vi "StartCAN.1.vi"(11 "CAN Interface":refnum<k21>="CAN1") -> (0 "error out":errorcluster, 1 "Tester Write Session out":refnum<k21>, 2 "Read Session out":refnum<k21>, 3 "DSC Write Session out":refnum<k21>)   [LabVIEW 2018]
uses:
  <vilib>/xnet/xnet.llb/XNET CAN Comm State.ctl
  <vilib>/xnet/xnet.llb/XNET Control Scope.ctl
  <vilib>/xnet/xnet.llb/XNET Frame CAN.ctl
  <vilib>/xnet/xnet.llb/XNET Frame Type CAN.ctl
  <vilib>/xnet/xnet.llb/XNET Create Session (Frame Input Queued).vi
  <vilib>/xnet/xnet.llb/XNET Create Session (Frame Output Single-point).vi
  <vilib>/xnet/xnet.llb/XNET Read (State CAN Comm).vi
  <vilib>/xnet/xnet.llb/XNET Wait (Interface Communicating).vi
  <resource>/objmgr/xnet.rc
  <vilib>/xnet/xnet.llb/XNET Write (Frame CAN).vi
panel:
  in  "error in (no error)":errorcluster
  out "TesterPresentSession":refnum<k21>
  out "CAN:I/O Mode":u32(ring) items=["CAN 2.0", "CAN FD", "CAN FD+BRS"]
  out "Protocol":u32(ring) items=["CAN", "FlexRay", "LIN"]
  out "CAN:Transceiver Capability":u32(ring) items=["HS"=0, "LS"=1, "XS"=3, "XS (HS/LS)"=4]
  out "Interface:CAN:Transceiver State":u32(ring) items=["Normal", "Sleep", "Single Wire Wakeup", "Single Wire High-Speed"]
  out "Interface:CAN:Transceiver State 2":u32(ring) items=["Normal", "Sleep", "Single Wire Wakeup", "Single Wire High-Speed"]
  out "Interface:CAN:Transceiver State 3":u32(ring) items=["Normal", "Sleep", "Single Wire Wakeup", "Single Wire High-Speed"]
  out "CAN:Termination Capability":u32(ring) items=["No", "Yes"]
  out "Array":T1[](array[typedef]) items=["Error Active", "Error Passive", "Bus Off", "Init"]
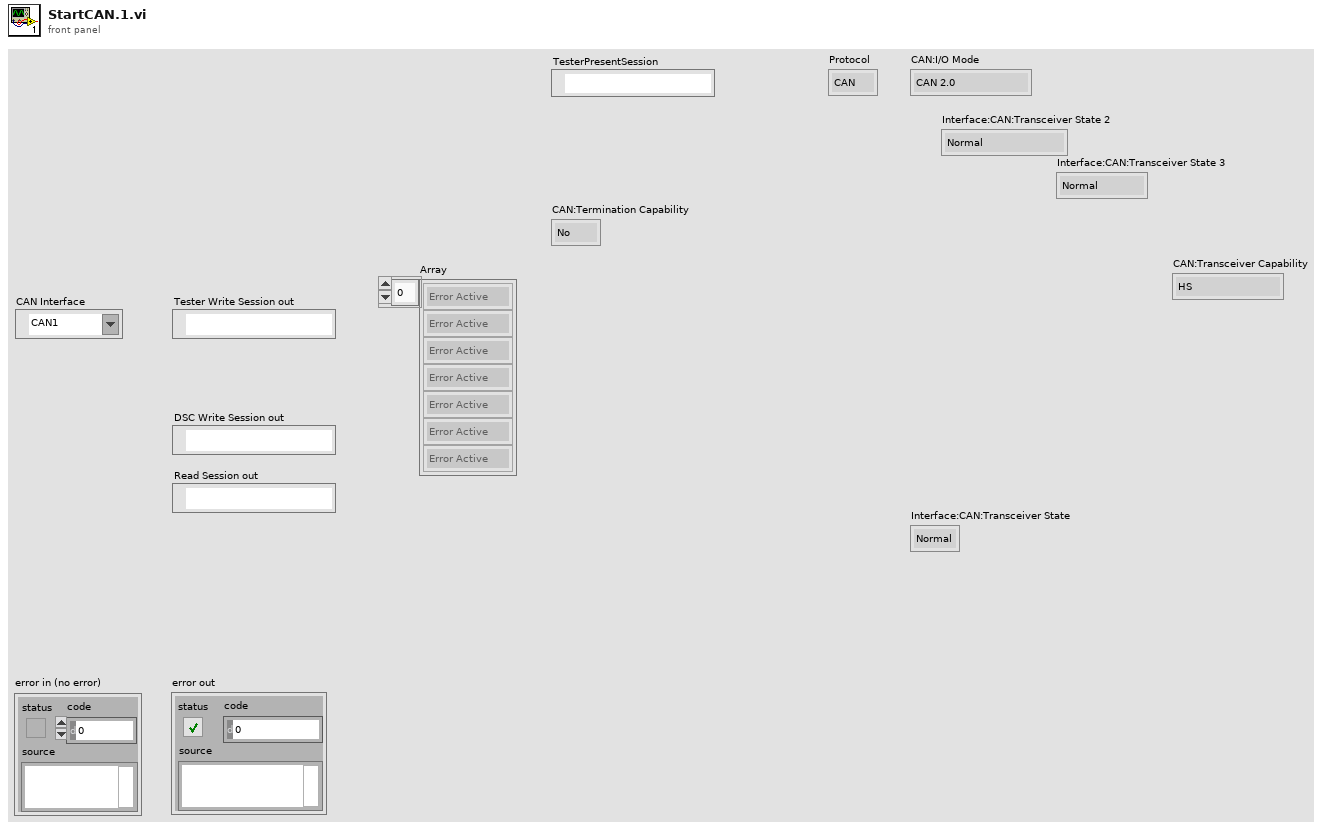
[diagram p1: front panel]
types:
  T1 = typedef "XNET CAN Comm State.ctl" = u8
  T2 = cluster{"Comment":string, "Default Payload":u8[], "Identifier":u32, "Name (Short)":string, "Payload Length":u32, "PDU_Mapping":cluster{"PDU":string, "Start Bit":u32, "Update Bit":i32}[], "CAN:Extended Identifier?":bool, "CAN:Timing Type":u32, "CAN:Transmit Time":dbl, "CAN:I/O Mode":u32}
  T3 = typedef "XNET Frame CAN.ctl" = cluster{"timestamp":timestamp, "payload":u8[], "identifier":u32, "type":T4, "extended?":bool, "echo?":bool}
  T4 = typedef "XNET Frame Type CAN.ctl" = u8
  T5 = typedef "XNET Control Scope.ctl" = u32
  T6 = typedef "XNET CAN Comm.ctl" = cluster{"fault code":i32, "fault?":bool, "communication state":T1, "last error":T7, "receive error counter":u8, "transmit error counter":u8, "transceiver error?":bool, "sleep?":bool}
  T7 = typedef "XNET CAN Last Err.ctl" = u8
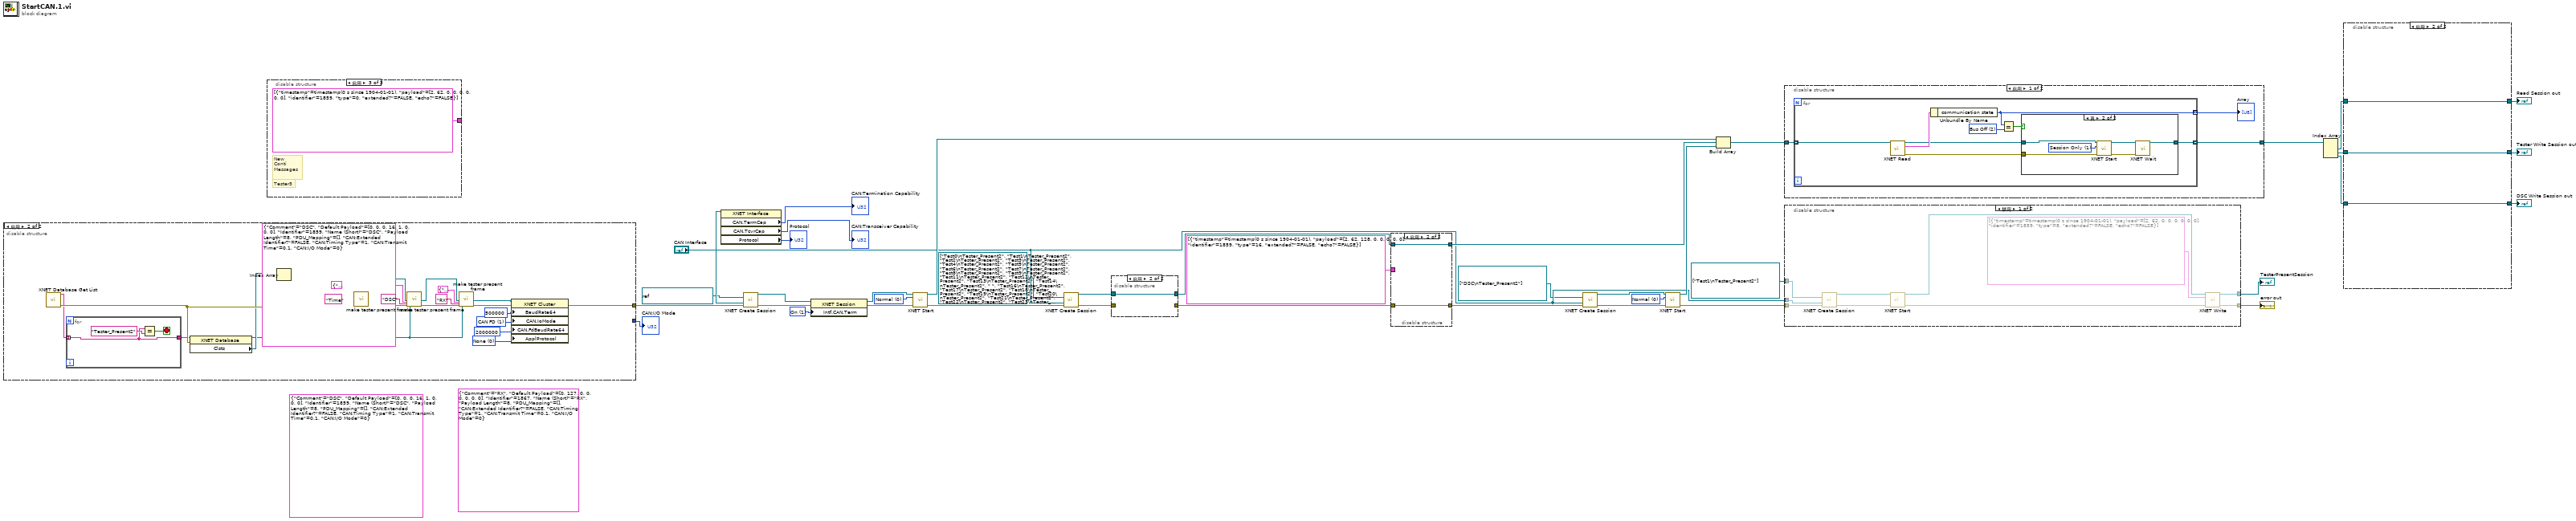
[diagram p0: block diagram]
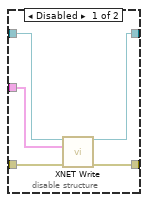
[diagram p2: hidden frame]
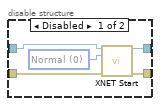
[diagram p3: hidden frame]
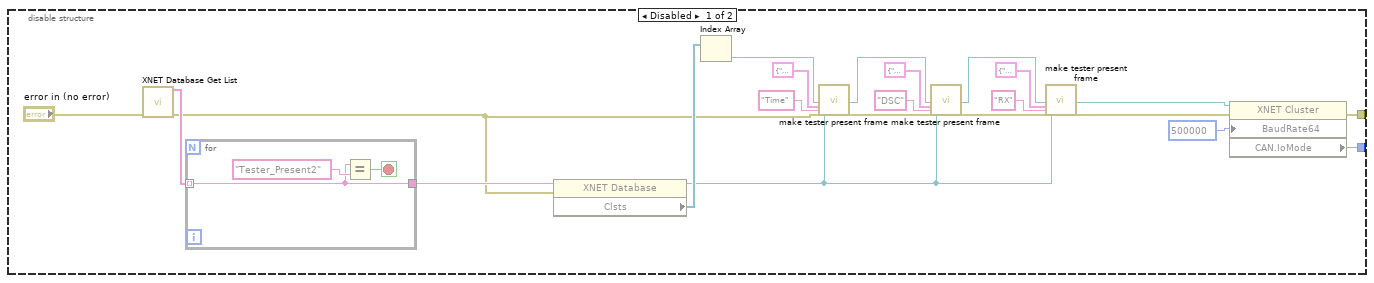
[diagram p4: hidden frame]
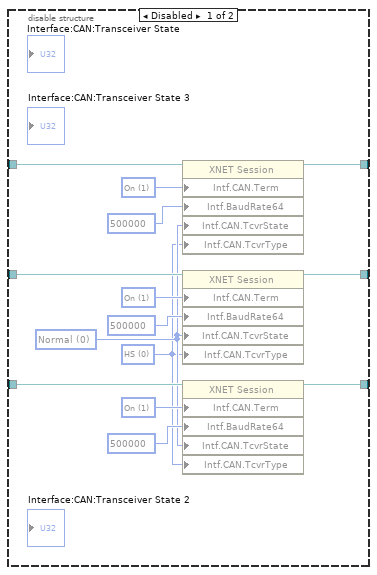
[diagram p6: hidden frame]
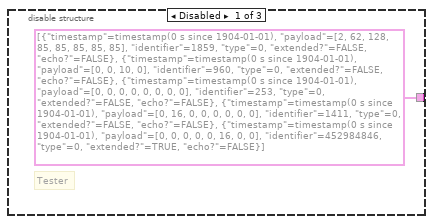
[diagram p9: hidden frame]
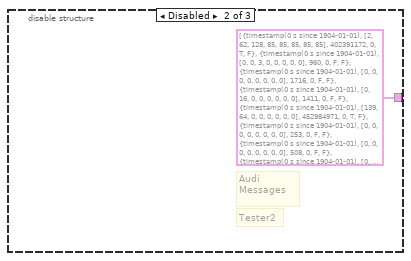
[diagram p10: hidden frame]
diagram:
  (unwired) T2 {"Comment"="DSC", "Default Payload"=[0, 0, 0, 16, 1, 0, 0, 0], "Identifier"=1859, "Name (Short)"="DSC", "Payload Length"=8, "PDU_Mapping"=[], "CAN:Extended Identifier?"=FALSE, "CAN:Timing Type"=1, "CAN:Transmit Time"=0.1, "CAN:I/O Mode"=0} ("New Frame Properties")
  (unwired) T2 {"Comment"="RX", "Default Payload"=[0, 127, 0, 0, 0, 0, 0, 0], "Identifier"=1867, "Name (Short)"="RX", "Payload Length"=8, "PDU_Mapping"=[], "CAN:Extended Identifier?"=FALSE, "CAN:Timing Type"=1, "CAN:Transmit Time"=0.1, "CAN:I/O Mode"=0} ("New Frame Properties")
  w11 = u32 1 items=["Off", "On"] ("Interface:CAN:Termination")
  w29 = T5 0 items=["Normal", "Session Only", "Interface Only", "Session Only Blocking"] ("scope (normal)")
  w30 = T5 0 items=["Normal", "Session Only", "Interface Only", "Session Only Blocking"] ("scope (normal)")
  n1 = disable-structure shown="启用" {
    disable-tunnel: [w60 w69] -> w40
    disable-tunnel: [w41 _] -> w15
    frame Disabled {
      n2 = call <vilib>:"XNET Database Get List.vi"("error in (no error)"="error in (no error)") -> ("array of alias"=w50:string[], "error out"=w46:errorcluster)  [unwired: 12 in, 1 out]
      n3 = for {
        tunnel: w50 -> [w63] mode=indexing
        tunnel: [w63] -> w49
        stop <- w64 stop-if-true
        n4 = Equal?(x=w63, y="Tester_Present2") -> (x = y?=w64:bool)
      }
      n5 = property class="XNET Database"(reference=w49, error in=w46) -> (reference out=w42:refnum<k21>, "Clsts"=w61:refnum<k21>[])  [unwired: 1 out]
      n6 = Index Array(array=w61) -> (element=w44:refnum<k21>)  [unwired: 1 in]
      n7 = call "make tester present frame.vi"("Cluster::"=w44, "New Frame Properties"=T2 {"Comment"="DSC", "Default Payload"=[0, 0, 0, 0, 0, 0, 0, 0], "Identifier"=1714, "Name (Short)"="Time", "Payload Length"=8, "PDU_Mapping"=[], "CAN:Extended Identifier?"=FALSE, "CAN:Timing Type"=0, "CAN:Transmit Time"=0.001, "CAN:I/O Mode"=0}, "frame name"="Time", "error in (no error)"=w46, "database in"=w42) -> ("target cluster out"=w43:refnum<k21>, "error out"=w45:errorcluster)  [unwired: 21 in]
      n8 = call "make tester present frame.vi"("Cluster::"=w43, "New Frame Properties"=T2 {"Comment"="DSC", "Default Payload"=[0, 0, 0, 0, 0, 0, 0, 0], "Identifier"=402391172, "Name (Short)"="DSC", "Payload Length"=8, "PDU_Mapping"=[], "CAN:Extended Identifier?"=TRUE, "CAN:Timing Type"=1, "CAN:Transmit Time"=0.001, "CAN:I/O Mode"=0}, "frame name"="DSC", "error in (no error)"=w45, "database in"=w42) -> ("target cluster out"=w59:refnum<k21>, "error out"=w58:errorcluster)  [unwired: 21 in]
      n9 = call "make tester present frame.vi"("Cluster::"=w59, "New Frame Properties"=T2 {"Comment"="RX", "Default Payload"=[0, 127, 0, 0, 0, 0, 0, 0], "Identifier"=402522244, "Name (Short)"="RX", "Payload Length"=8, "PDU_Mapping"=[], "CAN:Extended Identifier?"=TRUE, "CAN:Timing Type"=1, "CAN:Transmit Time"=0.001, "CAN:I/O Mode"=0}, "frame name"="RX", "error in (no error)"=w58, "database in"=w42) -> ("target cluster out"=w52:refnum<k21>, "error out"=w51:errorcluster)  [unwired: 21 in]
      n10 = property class="XNET Cluster"(reference=w52, error in=w51, "BaudRate64"=u64 500000 ("64bit Baud Rate")) -> (error out=w60:errorcluster, "CAN.IoMode"=w41:u32)  [unwired: 1 out]
    }
    frame Enabled {
      w66 = u32 0 items=["None", "J1939"] ("Application Protocol")
      w68 = u32 1 items=["CAN 2.0", "CAN FD", "CAN FD+BRS"] ("CAN:I/O Mode")
      n11 = call <vilib>:"XNET Database Get List.vi"() -> ("array of alias"=w85:string[], "error out"=w86:errorcluster)  [unwired: 13 in, 1 out]
      n12 = for {
        tunnel: w85 -> [w89] mode=indexing
        tunnel: [w89] -> w72
        stop <- w90 stop-if-true
        n13 = Equal?(x=w89, y="Tester_Present2") -> (x = y?=w90:bool)
      }
      n14 = property class="XNET Database"(reference=w72, error in=w86) -> (reference out=w71:refnum<k21>, "Clsts"=w73:refnum<k21>[])  [unwired: 1 out]
      n15 = Index Array(array=w73) -> (element=w88:refnum<k21>)  [unwired: 1 in]
      n16 = call "make tester present frame.vi"("Cluster::"=w88, "New Frame Properties"=T2 {"Comment"="Time", "Default Payload"=[0, 0, 0, 0, 0, 0, 0, 0], "Identifier"=1859, "Name (Short)"="Time", "Payload Length"=8, "PDU_Mapping"=[], "CAN:Extended Identifier?"=FALSE, "CAN:Timing Type"=0, "CAN:Transmit Time"=0.1, "CAN:I/O Mode"=0}, "frame name"="Time", "error in (no error)"=w86, "database in"=w71) -> ("target cluster out"=w70:refnum<k21>, "error out"=w87:errorcluster)  [unwired: 21 in]
      n17 = call "make tester present frame.vi"("Cluster::"=w70, "New Frame Properties"=T2 {"Comment"="DSC", "Default Payload"=[0, 0, 0, 16, 1, 0, 0, 0], "Identifier"=1859, "Name (Short)"="DSC", "Payload Length"=8, "PDU_Mapping"=[], "CAN:Extended Identifier?"=FALSE, "CAN:Timing Type"=1, "CAN:Transmit Time"=0.1, "CAN:I/O Mode"=0}, "frame name"="DSC", "error in (no error)"=w87, "database in"=w71) -> ("target cluster out"=w81:refnum<k21>, "error out"=w82:errorcluster)  [unwired: 21 in]
      n18 = call "make tester present frame.vi"("Cluster::"=w81, "New Frame Properties"=T2 {"Comment"="RX", "Default Payload"=[0, 0, 0, 0, 0, 0, 0, 0], "Identifier"=1867, "Name (Short)"="RX", "Payload Length"=8, "PDU_Mapping"=[], "CAN:Extended Identifier?"=FALSE, "CAN:Timing Type"=1, "CAN:Transmit Time"=0.001, "CAN:I/O Mode"=1}, "frame name"="RX", "error in (no error)"=w82, "database in"=w71) -> ("target cluster out"=w83:refnum<k21>, "error out"=w84:errorcluster)  [unwired: 21 in]
      n19 = property class="XNET Cluster"(reference=w83, error in=w84, "BaudRate64"=u64 500000 ("64bit Baud Rate"), "CAN.IoMode"=w68, "CAN.FdBaudRate64"=u64 2000000 ("CAN:64bit FD Baud Rate"), "ApplProtocol"=w66) -> (error out=w69:errorcluster)  [unwired: 1 out]
    }
  }
  "CAN:I/O Mode" <- w15
  n20 = disable-structure shown="启用" {
    disable-tunnel: [T3[] [{"timestamp"=timestamp(0 s since 1904-01-01), "payload"=[2, 62, 128, 85, 85, 85, 85, 85], "identifier"=1859, "type"=0, "extended?"=FALSE, "echo?"=FALSE}, {"timestamp"=timestamp(0 s since 1904-01-01), "payload"=[0, 0, 10, 0], "identifier"=960, "type"=0, "extended?"=FALSE, "echo?"=FALSE}, {"timestamp"=timestamp(0 s since 1904-01-01), "payload"=[0, 0, 0, 0, 0, 0, 0, 0], "identifier"=253, "type"=0, "extended?"=FALSE, "echo?"=FALSE}, {"timestamp"=timestamp(0 s since 1904-01-01), "payload"=[0, 16, 0, 0, 0, 0, 0, 0], "identifier"=1411, "type"=0, "extended?"=FALSE, "echo?"=FALSE}, {"timestamp"=timestamp(0 s since 1904-01-01), "payload"=[0, 0, 0, 0, 0, 16, 0, 0], "identifier"=452984846, "type"=0, "extended?"=TRUE, "echo?"=FALSE}] ("data") T3[] [{"timestamp"=timestamp(0 s since 1904-01-01), "payload"=[2, 62, 128, 85, 85, 85, 85, 85], "identifier"=402391172, "type"=0, "extended?"=TRUE, "echo?"=FALSE}, {"timestamp"=timestamp(0 s since 1904-01-01), "payload"=[0, 0, 3, 0, 0, 0, 0, 0], "identifier"=960, "type"=0, "extended?"=FALSE, "echo?"=FALSE}, {"timestamp"=timestamp(0 s since 1904-01-01), "payload"=[0, 0, 0, 0, 0, 0, 0, 0], "identifier"=1716, "type"=0, "extended?"=FALSE, "echo?"=FALSE}, {"timestamp"=timestamp(0 s since 1904-01-01), "payload"=[0, 16, 0, 0, 0, 0, 0, 0], "identifier"=1411, "type"=0, "extended?"=FALSE, "echo?"=FALSE}, {"timestamp"=timestamp(0 s since 1904-01-01), "payload"=[139, 64, 0, 0, 0, 0, 0, 0], "identifier"=452984971, "type"=0, "extended?"=TRUE, "echo?"=FALSE}, {"timestamp"=timestamp(0 s since 1904-01-01), "payload"=[0, 0, 0, 0, 0, 0, 0, 0], "identifier"=253, "type"=0, "extended?"=FALSE, "echo?"=FALSE}, {"timestamp"=timestamp(0 s since 1904-01-01), "payload"=[0, 0, 0, 0, 0, 0, 0, 0], "identifier"=508, "type"=0, "extended?"=FALSE, "echo?"=FALSE}, {"timestamp"=timestamp(0 s since 1904-01-01), "payload"=[0, 0, 0, 0, 150, 0, 0, 0], "identifier"=1646, "type"=0, "extended?"=FALSE, "echo?"=FALSE}, {"timestamp"=timestamp(0 s since 1904-01-01), "payload"=[0, 0, 0, 0, 0, 0, 0, 150], "identifier"=1719, "type"=0, "extended?"=FALSE, "echo?"=FALSE}, {"timestamp"=timestamp(0 s since 1904-01-01), "payload"=[0, 0, 4, 0, 0, 0, 0, 0], "identifier"=958, "type"=0, "extended?"=FALSE, "echo?"=FALSE}, {"timestamp"=timestamp(0 s since 1904-01-01), "payload"=[0, 0, 0, 0, 0, 0, 0, 0], "identifier"=1635, "type"=0, "extended?"=FALSE, "echo?"=FALSE}, {"timestamp"=timestamp(0 s since 1904-01-01), "payload"=[0, 0, 0, 0, 0, 0, 0, 0], "identifier"=319, "type"=0, "extended?"=FALSE, "echo?"=FALSE}, {"timestamp"=timestamp(0 s since 1904-01-01), "payload"=[0, 0, 0, 0, 0, 0, 0, 0], "identifier"=1616, "type"=0, "extended?"=FALSE, "echo?"=FALSE}, {"timestamp"=timestamp(0 s since 1904-01-01), "payload"=[0, 12, 0, 0, 0, 0, 0, 0], "identifier"=1413, "type"=0, "extended?"=FALSE, "echo?"=FALSE}, {"timestamp"=timestamp(0 s since 1904-01-01), "payload"=[0, 0, 0, 0, 0, 0, 0, 0], "identifier"=1462, "type"=0, "extended?"=FALSE, "echo?"=FALSE}, {"timestamp"=timestamp(0 s since 1904-01-01), "payload"=[16, 64, 0, 0, 0, 16, 0, 0], "identifier"=452984848, "type"=0, "extended?"=TRUE, "echo?"=FALSE}, {"timestamp"=timestamp(0 s since 1904-01-01), "payload"=[0, 0, 0, 0, 0, 0, 0, 0], "identifier"=976, "type"=0, "extended?"=FALSE, "echo?"=FALSE}, {"timestamp"=timestamp(0 s since 1904-01-01), "payload"=[0, 0, 0, 0, 0, 0, 0, 0], "identifier"=974, "type"=0, "extended?"=FALSE, "echo?"=FALSE}, {"timestamp"=timestamp(0 s since 1904-01-01), "payload"=[74, 64, 0, 0, 0, 0, 0, 0], "identifier"=452984906, "type"=0, "extended?"=TRUE, "echo?"=FALSE}, {"timestamp"=timestamp(0 s since 1904-01-01), "payload"=[0, 0, 0, 0, 0, 0, 0, 0], "identifier"=977, "type"=0, "extended?"=FALSE, "echo?"=FALSE}, {"timestamp"=timestamp(0 s since 1904-01-01), "payload"=[0, 0, 0, 0, 0, 0, 0, 0], "identifier"=975, "type"=0, "extended?"=FALSE, "echo?"=FALSE}, {"timestamp"=timestamp(0 s since 1904-01-01), "payload"=[75, 64, 0, 0, 0, 0, 0, 0], "identifier"=452984907, "type"=0, "extended?"=TRUE, "echo?"=FALSE}] ("Array 3") T3[] [{"timestamp"=timestamp(0 s since 1904-01-01), "payload"=[2, 62, 0, 0, 0, 0, 0, 0], "identifier"=1859, "type"=0, "extended?"=FALSE, "echo?"=FALSE}] ("data")] -> _
    frame Disabled {
      # "Tester"
    }
    frame Disabled {
      # "Tester2"
      # "Audi\nMessages"
    }
    frame Enabled {
      # "Tester3"
      # "New\nConti\nMessages"
    }
  }
  n21 = property class="XNET Interface"(reference="CAN Interface") -> ("CAN.TermCap"=→"CAN:Termination Capability":u32, "CAN.TcvrCap"=→"CAN:Transceiver Capability":u32, "Protocol"=→"Protocol":u32)  [unwired: 1 in, 2 out]
  n22 = call-poly <vilib>:"XNET Create Session.vi"("frame"=refnum<k21> "RX\nTester_Present2" ("XNET Frame"), "interface"="CAN Interface", "error in (no error)"=w40) -> ("session out"=w14:refnum<k21>, "error out"=w12:errorcluster)  [unwired: 11 in]
  n23 = property class="XNET Session"(reference=w14, error in=w12, "Intf.CAN.Term"=w11) -> (reference out=w13:refnum<k21>, error out=w10:errorcluster)
  n24 = call <vilib>:"XNET Start.vi"("session in"=w13, "scope (normal)"=w30, "error in (no error)"=w10) -> ("session out"=w37:refnum<k21>, "error out"=w32:errorcluster)  [unwired: 11 in]
  n25 = call-poly <vilib>:"XNET Create Session.vi"("frame list"=refnum<k21>[] ["Test0\nTester_Present2", "Test1\nTester_Present2", "Test2\nTester_Present2", "Test3\nTester_Present2", "Test4\nTester_Present2", "Test5\nTester_Present2", "Test6\nTester_Present2", "Test7\nTester_Present2", "Test8\nTester_Present2", "Test9\nTester_Present2", "Test11\nTester_Present2", "Test12\nTester_Present2", "Test13\nTester_Present2", "Test14\nTester_Present2", " ", "Test16\nTester_Present2", "Test17\nTester_Present2", "Test18\nTester_Present2", "Test19\nTester_Present2", "Test20\nTester_Present2", "Test21\nTester_Present2", "Test22\nTester_Present2", "Test23\nTester_Present2", "Test24\nTester_Present2", "Test25\nTester_Present2", "Test26\nTester_Present2", "Test27\nTester_Present2"] ("Frames"), "interface"="CAN Interface", "error in (no error)"=w32) -> ("session out"=w27:refnum<k21>, "error out"=w28:errorcluster)  [unwired: 11 in]
  n26 = disable-structure shown="启用" {
    disable-tunnel: [w99 w100] -> w39
    disable-tunnel: [w98 _] -> w38
    disable-tunnel: w28 -> [w96 _]
    disable-tunnel: w27 -> [w95 w100]
    frame Disabled {
      w97 = T5 0 items=["Normal", "Session Only", "Interface Only", "Session Only Blocking"] ("scope (normal)")
      n27 = call <vilib>:"XNET Start.vi"("session in"=w95, "scope (normal)"=w97, "error in (no error)"=w96) -> ("session out"=w99:refnum<k21>, "error out"=w98:errorcluster)  [unwired: 11 in]
    }
    frame Enabled {
    }
  }
  n28 = disable-structure shown="启用" {
    disable-tunnel: w39 -> [w105 w106]
    disable-tunnel: w38 -> [w104 w107]
    disable-tunnel: [w103 w106] -> w36
    disable-tunnel: [w102 w107] -> w31
    disable-tunnel: T3[] [{"timestamp"=timestamp(0 s since 1904-01-01), "payload"=[2, 62, 128, 0, 0, 0, 0, 0], "identifier"=1859, "type"=16, "extended?"=FALSE, "echo?"=FALSE}] ("data") -> [w101 _]
    frame Disabled {
      n29 = call-poly <vilib>:"XNET Write.vi"("session in"=w105, "data"=w101, "error in (no error)"=w104) -> ("session out"=w103:refnum<k21>, "error out"=w102:errorcluster)  [unwired: 11 in]
    }
    frame Enabled {
    }
  }
  n30 = call-poly <vilib>:"XNET Create Session.vi"("frame list"=refnum<k21>[] ["DSC\nTester_Present2"] ("Frames"), "interface"="CAN Interface", "error in (no error)"=w31) -> ("session out"=w26:refnum<k21>, "error out"=w25:errorcluster)  [unwired: 11 in]
  n31 = call <vilib>:"XNET Start.vi"("session in"=w26, "scope (normal)"=w29, "error in (no error)"=w25) -> ("session out"=w35:refnum<k21>, "error out"=w6:errorcluster)  [unwired: 11 in]
  n32 = Build Array(w37, w36, w35) -> (w34:refnum<k21>[])
  n33 = disable-structure shown="启用" {
    disable-tunnel: w34 -> [w110 w126]
    disable-tunnel: [w108 w126] -> w33
    frame Enabled {
      n34 = for {
        tunnel: w110 -> [w117] mode=indexing
        tunnel: [w112] -> w109 mode=indexing
        tunnel: [w111] -> w108 mode=indexing
        w116 = T1 2 items=["Error Active", "Error Passive", "Bus Off", "Init"] ("y")
        n35 = call-poly <vilib>:"XNET Read.vi"("session in"=w117) -> ("session out"=w114:refnum<k21>, "CAN comm"=w118:T6, "error out"=w113:errorcluster)  [unwired: 12 in]
        n36 = Unbundle By Name(w118) -> ("communication state"=w112:T1)
        n37 = Equal?(x=w112, y=w116) -> (x = y?=w115:bool)
        n38 = case shown="真" w115 {
          tunnel: w114 -> [w119 w125]
          tunnel: w113 -> [_ w123]
          tunnel: [w119 w120] -> w111
          frame False {
          }
          frame True {
            w121 = T5 1 items=["Normal", "Session Only", "Interface Only", "Session Only Blocking"] ("scope (normal)")
            n39 = call <vilib>:"XNET Start.vi"("session in"=w125, "scope (normal)"=w121, "error in (no error)"=w123) -> ("session out"=w124:refnum<k21>, "error out"=w122:errorcluster)  [unwired: 11 in]
            n40 = call-poly <vilib>:"XNET Wait.vi"("session in"=w124, "error in (no error)"=w122) -> ("session out"=w120:refnum<k21>)  [unwired: 12 in, 1 out]
          }
        }
      }
      "Array" <- w109
    }
    frame Disabled {
    }
  }
  n41 = disable-structure shown="禁用" {
    disable-tunnel: "CAN Interface" -> [w136 _]
    disable-tunnel: [w128 _] -> w8
    disable-tunnel: [w129 _] -> w7
    disable-tunnel: refnum<k21>[] ["Test1\nTester_Present2"] ("Frames") -> [w135 _]
    disable-tunnel: w6 -> [w132 _]
    frame Disabled {
      n42 = call-poly <vilib>:"XNET Create Session.vi"("frame list"=w135, "interface"=w136, "error in (no error)"=w132) -> ("session out"=w134:refnum<k21>, "error out"=w133:errorcluster)  [unwired: 11 in]
      n43 = call <vilib>:"XNET Start.vi"("session in"=w134, "error in (no error)"=w133) -> ("session out"=w131:refnum<k21>, "error out"=w130:errorcluster)  [unwired: 12 in]
      n44 = call-poly <vilib>:"XNET Write.vi"("session in"=w131, "data"=T3[] [{"timestamp"=timestamp(0 s since 1904-01-01), "payload"=[2, 62, 0, 0, 0, 0, 0, 0], "identifier"=1859, "type"=8, "extended?"=FALSE, "echo?"=FALSE}], "error in (no error)"=w130) -> ("session out"=w128:refnum<k21>, "error out"=w129:errorcluster)  [unwired: 11 in]
    }
    frame Enabled {
    }
  }
  "error out" <- w7
  "TesterPresentSession" <- w8
  n45 = Index Array(array=w33) -> (element #1=w23:refnum<k21>, element #2=w21:refnum<k21>, element #3=w19:refnum<k21>)  [unwired: 3 in]
  n46 = disable-structure shown="启用" {
    disable-tunnel: w23 -> [w149 w153]
    disable-tunnel: [w148 w153] -> w22
    disable-tunnel: w21 -> [w145 w152]
    disable-tunnel: [w144 w152] -> w20
    disable-tunnel: w19 -> [w143 w151]
    disable-tunnel: [w142 w151] -> w18
    frame Disabled {
      w137 = u32 0 items=["HS", "LS", "SW", "Ext", "Disc"] ("Interface:CAN:Transceiver Type")
      w138 = u32 0 items=["Normal", "Sleep", "Single Wire Wakeup", "Single Wire High-Speed"] ("Interface:CAN:Transceiver State")
      w146 = u32 1 items=["Off", "On"] ("Interface:CAN:Termination")
      w147 = u32 1 items=["Off", "On"] ("Interface:CAN:Termination")
      w150 = u32 1 items=["Off", "On"] ("Interface:CAN:Termination")
      n47 = property class="XNET Session"(reference=w149, "Intf.CAN.Term"=w150, "Intf.BaudRate64"=u64 500000 ("Interface:64bit Baud Rate"), "Intf.CAN.TcvrState"=w138, "Intf.CAN.TcvrType"=w137) -> (reference out=w148:refnum<k21>)  [unwired: 1 in, 1 out]
      n48 = property class="XNET Session"(reference=w145, "Intf.CAN.Term"=w147, "Intf.BaudRate64"=u64 500000 ("Interface:64bit Baud Rate"), "Intf.CAN.TcvrState"=w138, "Intf.CAN.TcvrType"=w137) -> (reference out=w144:refnum<k21>)  [unwired: 1 in, 1 out]
      n49 = property class="XNET Session"(reference=w143, "Intf.CAN.Term"=w146, "Intf.BaudRate64"=u64 500000 ("Interface:64bit Baud Rate"), "Intf.CAN.TcvrState"=w138, "Intf.CAN.TcvrType"=w137) -> (reference out=w142:refnum<k21>)  [unwired: 1 in, 1 out]
    }
    frame Enabled {
    }
  }
  "Tester Write Session out" <- w20
  "Read Session out" <- w22
  "DSC Write Session out" <- w18
